vi "LV2010_rshmc804x_SimpleExample_original.vi"() -> ()   [LabVIEW 2010]
uses:
  <instrlib>/Rohde&Schwarz HMC 804x Power Supplies/Rohde&Schwarz HMC 804x Power Supplies.lvlib
panel:
  out "Screenshot":picture
  in  "CH2 Current":dbl=2.2
  in  "CH1 Current":dbl=1.1
  in  "CH1 enabled":bool caption="CH1 ON"
  in  "CH2 enabled":bool caption="CH2 ON"
  in  "CH2 Voltage":dbl=5.0
  in  "CH1 Voltage":dbl=3.0
  # "HMC804x simple example"
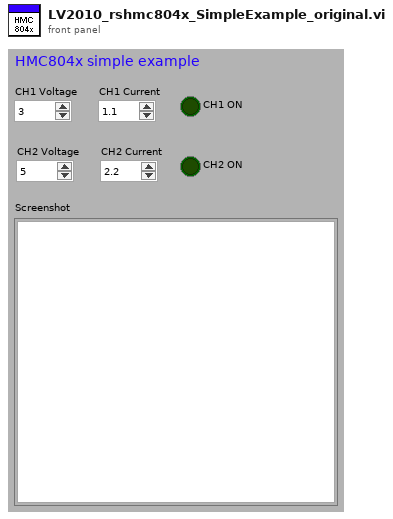
[diagram p1: front panel]
types:
  T1 = typedef "imagedata.ctl" = cluster{"image type":i32, "image depth":i32, "image":u8[], "mask":u8[], "colors":u32[], "Rectangle":cluster{"left":i16, "top":i16, "right":i16, "bottom":i16}}
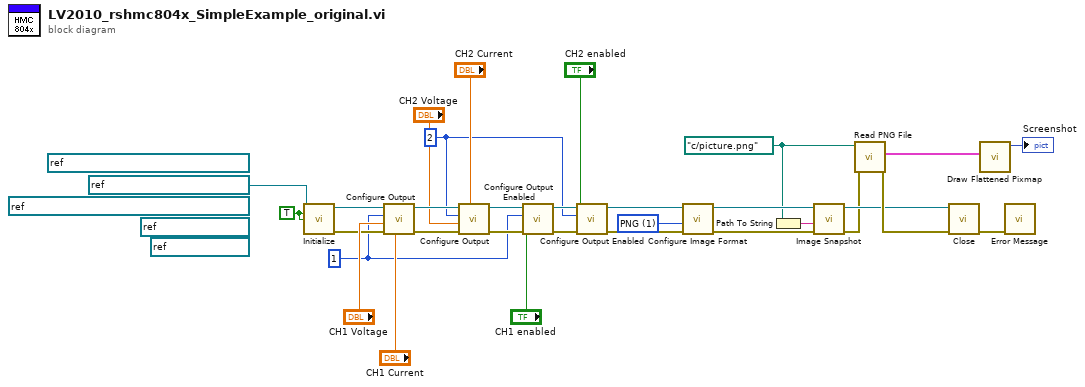
[diagram p0: block diagram]
diagram:
  w3 = path "c:/picture.png" ("path to BMP file")
  w6 = 1 items=["BMP", "PNG"] ("Image Format (BMP)")
  (unwired) refnum<visa-resource-name> "TCPIP::10.85.0.106::5025::SOCKET" ("VISA resource name")
  (unwired) refnum<visa-resource-name> "ASRL5::INSTR" ("VISA resource name")
  w15 = TRUE ("ID Query (T: Check)")
  (unwired) refnum<visa-resource-name> "GPIB::12::INSTR" ("VISA resource name")
  w18 = 2 ("Channel (1)")
  w21 = 1 ("Channel (1)")
  (unwired) refnum<visa-resource-name> "USB0::0x0AAD::0x0135::000000000::INSTR" ("VISA resource name")
  n1 = call <instrlib>:"Initialize.vi"("VISA resource name"=refnum<visa-resource-name> "TCPIP::10.85.0.114::INSTR", "ID Query (T: Check)"=w15, "Reset (T: Reset)"=w15) -> ("VISA resource name out"=w28:refnum<visa-resource-name>, "error out"=w27:errorcluster)  [unwired: 11 in]
  n2 = call <instrlib>:"Configure Output.vi"("Current (0.0)"="CH1 Current", "error in (no error)"=w27, "Voltage (0.0)"="CH1 Voltage", "Channel (1)"=w21, "VISA resource name"=w28) -> ("error out"=w25:errorcluster, "VISA resource name out"=w26:refnum<visa-resource-name>)  [unwired: 5 in]
  n3 = call <instrlib>:"Configure Output.vi"("Current (0.0)"="CH2 Current", "error in (no error)"=w25, "Voltage (0.0)"="CH2 Voltage", "Channel (1)"=w18, "VISA resource name"=w26) -> ("error out"=w23:errorcluster, "VISA resource name out"=w22:refnum<visa-resource-name>)  [unwired: 5 in]
  n4 = call <instrlib>:"Configure Output Enabled.vi"("error in (no error)"=w23, "Enabled (Off)"="CH1 enabled", "Channel (1)"=w21, "VISA resource name"=w22) -> ("error out"=w19:errorcluster, "VISA resource name out"=w20:refnum<visa-resource-name>)  [unwired: 6 in]
  n5 = call <instrlib>:"Configure Output Enabled.vi"("error in (no error)"=w19, "Enabled (Off)"="CH2 enabled", "Channel (1)"=w18, "VISA resource name"=w20) -> ("error out"=w2:errorcluster, "VISA resource name out"=w1:refnum<visa-resource-name>)  [unwired: 6 in]
  n6 = call <instrlib>:"Configure Image Format.vi"("error in (no error)"=w2, "Image Format (BMP)"=w6, "VISA resource name"=w1) -> ("error out"=w7:errorcluster, "VISA resource name out"=w8:refnum<visa-resource-name>)  [unwired: 7 in]
  n7 = Path To String(path=w3) -> (string=w5:string)
  n8 = call <instrlib>:"Image Snapshot.vi"("error in (no error)"=w7, "Destination (\"\")"=w5, "VISA resource name"=w8) -> ("error out"=w4:errorcluster, "VISA resource name out"=w11:refnum<visa-resource-name>)  [unwired: 7 in]
  n9 = call <vilib>:"Read PNG File.vi"("error in (no error)"=w4, "path to PNG file"=w3) -> ("error out"=w12:errorcluster, "image data"=w14:T1)  [unwired: 7 in, 1 out]
  n10 = call <instrlib>:"Close.vi"("error in (no error)"=w12, "VISA resource name"=w11) -> ("error out"=w10:errorcluster)  [unwired: 9 in]
  n11 = call <vilib>:"Draw Flattened Pixmap.vi"("image data"=w14) -> ("new picture"=→"Screenshot":picture)  [unwired: 8 in]
  n12 = call <instrlib>:"Error Message.vi"("error in (no error)"=w10) -> ()  [unwired: 10 in, 5 out]
